vi "NeueSP.vi"(4 "Anzahl2":i32, 5 "Anzahl1":i32, 6 "AlteSP":dbl[](array[numeric]), 7 "NeueSP":dbl[](array[numeric]), 9 "BefehleCluster":T1, 10 "NeueSP":bool, 11 "ClusterFest":T2) -> (3 "BefehleCluster":T1)   [LabVIEW 2010]
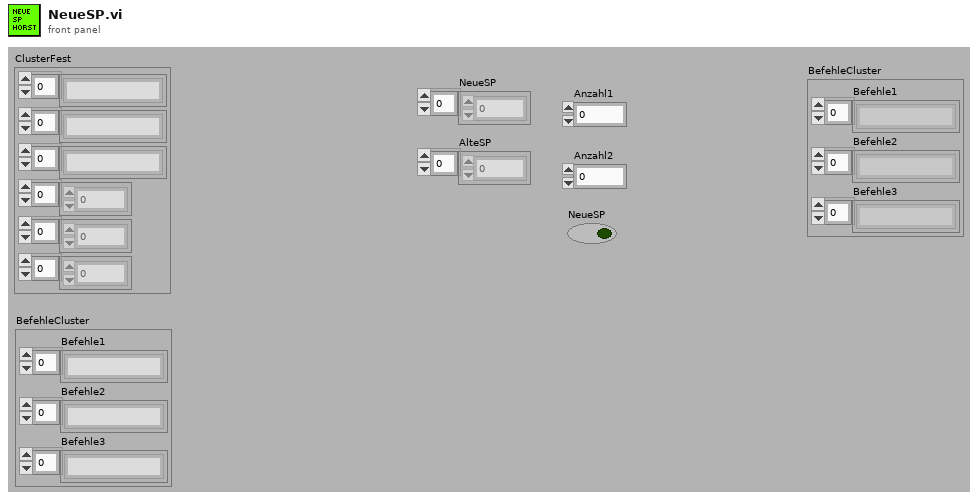
[diagram p1: front panel]
types:
  T1 = cluster{"Befehle1":string[], "Befehle2":string[], "Befehle3":string[]}
  T2 = cluster{string[], string[], string[], dbl[], dbl[], dbl[]}
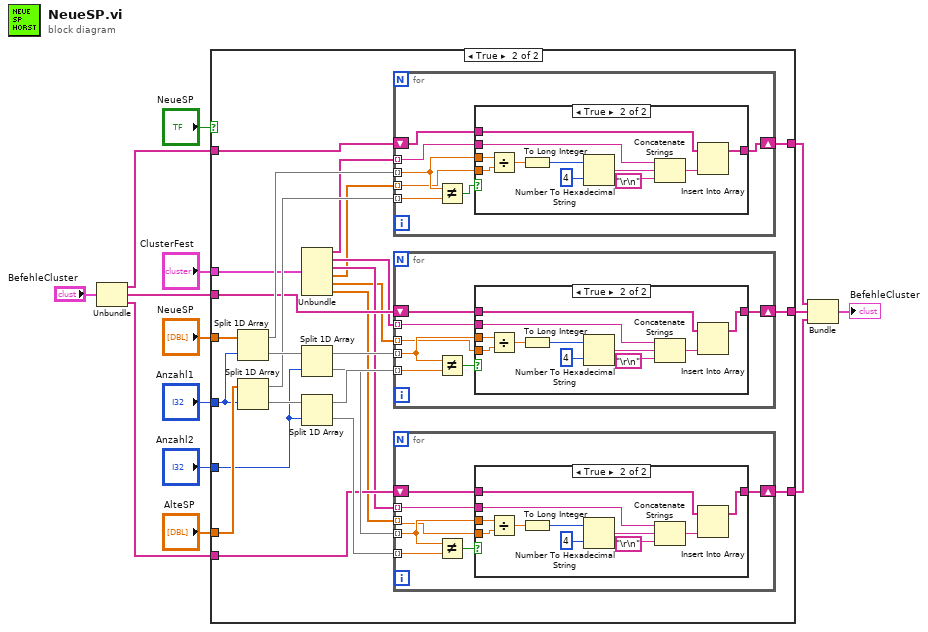
[diagram p0: block diagram]
diagram:
  n1 = Unbundle("BefehleCluster") -> ("Befehle1"=w3:string[], "Befehle2"=w2:string[], "Befehle3"=w1:string[])
  n2 = case shown="True" "NeueSP" {
    tunnel: "NeueSP" -> [_ w42]
    tunnel: "AlteSP" -> [_ w40]
    tunnel: w3 -> [w17 w32]
    tunnel: w2 -> [w16 w31]
    tunnel: w1 -> [w15 w30]
    tunnel: [w17 w29] -> w8
    tunnel: [w16 w26] -> w7
    tunnel: [w15 w25] -> w6
    tunnel: "Anzahl1" -> [_ w28]
    tunnel: "Anzahl2" -> [_ w27]
    tunnel: "ClusterFest" -> [_ w24]
    frame False {
    }
    frame True {
      n3 = Split 1D Array(array=w42, index=w28) -> (first subarray=w38:dbl[], second subarray=w41:dbl[])
      n4 = Split 1D Array(array=w40, index=w28) -> (first subarray=w37:dbl[], second subarray=w39:dbl[])
      n5 = Unbundle(w24) -> (w23:string[], w22:string[], w21:string[], w20:dbl[], w19:dbl[], w18:dbl[])
      n6 = Split 1D Array(array=w41, index=w27) -> (first subarray=w36:dbl[], second subarray=w34:dbl[])
      n7 = Split 1D Array(array=w39, index=w27) -> (first subarray=w35:dbl[], second subarray=w33:dbl[])
      n8 = for {
        tunnel: w38 -> [w83] mode=indexing
        tunnel: w37 -> [w87] mode=indexing
        shift-right: [w84] -> w29
        shift-left: w32 -> [w85]
        tunnel: w23 -> [w82] mode=indexing
        tunnel: w20 -> [w81] mode=indexing
        n9 = Not Equal?(x=w83, y=w87) -> (x != y?=w86:bool)
        n10 = case shown="True" w86 {
          tunnel: w85 -> [w88 w99]
          tunnel: [w88 w98] -> w84
          tunnel: w83 -> [_ w92]
          tunnel: w82 -> [_ w90]
          tunnel: w81 -> [_ w89]
          frame False {
          }
          frame True {
            n11 = Divide(x=w92, y=w89) -> (x/y=w97:dbl)
            n12 = To Long Integer(number=w97) -> (32bit integer=w96:i32)
            n13 = Number To Hexadecimal String(1:i16 4 ("Breite (-)"), 2:w96) -> (0:w94:string)
            n14 = Concatenate Strings(w90, w94, "\r\n") -> (w91:string)
            n15 = Insert Into Array(array=w99, new element=w91) -> (w98:string[])  [unwired: 1 in]
          }
        }
      }
      n16 = for {
        tunnel: w36 -> [w68] mode=indexing
        tunnel: w35 -> [w67] mode=indexing
        tunnel: w22 -> [w63] mode=indexing
        tunnel: w19 -> [w65] mode=indexing
        shift-right: [w62] -> w26
        shift-left: w31 -> [w64]
        n17 = Not Equal?(x=w68, y=w67) -> (x != y?=w66:bool)
        n18 = case shown="True" w66 {
          tunnel: w64 -> [w69 w80]
          tunnel: [w69 w79] -> w62
          tunnel: w68 -> [_ w73]
          tunnel: w63 -> [_ w71]
          tunnel: w65 -> [_ w70]
          frame False {
          }
          frame True {
            n19 = Divide(x=w73, y=w70) -> (x/y=w78:dbl)
            n20 = To Long Integer(number=w78) -> (32bit integer=w77:i32)
            n21 = Number To Hexadecimal String(1:i16 4 ("Breite (-)"), 2:w77) -> (0:w75:string)
            n22 = Concatenate Strings(w71, w75, "\r\n") -> (w72:string)
            n23 = Insert Into Array(array=w80, new element=w72) -> (w79:string[])  [unwired: 1 in]
          }
        }
      }
      n24 = for {
        tunnel: w34 -> [w46] mode=indexing
        tunnel: w33 -> [w49] mode=indexing
        tunnel: w21 -> [w44] mode=indexing
        tunnel: w18 -> [w45] mode=indexing
        shift-right: [w43] -> w25
        shift-left: w30 -> [w47]
        n25 = Not Equal?(x=w46, y=w49) -> (x != y?=w48:bool)
        n26 = case shown="True" w48 {
          tunnel: w47 -> [w50 w61]
          tunnel: [w50 w60] -> w43
          tunnel: w46 -> [_ w54]
          tunnel: w44 -> [_ w52]
          tunnel: w45 -> [_ w51]
          frame False {
          }
          frame True {
            n27 = Divide(x=w54, y=w51) -> (x/y=w59:dbl)
            n28 = To Long Integer(number=w59) -> (32bit integer=w58:i32)
            n29 = Number To Hexadecimal String(1:i16 4 ("Breite (-)"), 2:w58) -> (0:w56:string)
            n30 = Concatenate Strings(w52, w56, "\r\n") -> (w53:string)
            n31 = Insert Into Array(array=w61, new element=w53) -> (w60:string[])  [unwired: 1 in]
          }
        }
      }
    }
  }
  n32 = Bundle("Befehle1"=w8, "Befehle2"=w7, "Befehle3"=w6) -> (→"BefehleCluster":T1)  [unwired: 1 in]
